vi "配置文件路径.vi"() -> (3 "appended path":path)   [LabVIEW 2016, in "斯坦道CODCr.lvlib"]
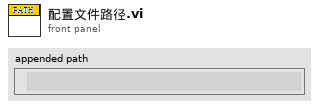
[diagram p1: front panel]
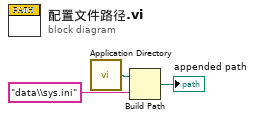
[diagram p0: block diagram]
diagram:
  n1 = call <vilib>:"Application Directory.vi"() -> ("Application Directory"=w2:path)
  n2 = Build Path(base path=w2, name or relative path="data\\sys.ini" ("名称或相对路径")) -> (appended path=→"appended path":path)
